vi "Listen.vi"(6 "Error":errorcluster, 7 "Actor":refnum<class "Actor Layer.lvclass">, 10 "Msg DVR":refnum<data-value>, 11 "Actor":T1) -> (3 "Actor":T1, 4 "Error":errorcluster, 5 "Actor":refnum<class "Actor Layer.lvclass">)   [LabVIEW 2020, in "jettl.lvlib"]
uses:
  jettl.lvlib
  Msg/Msg.lvclass
  Actor Layer/Actor Layer.lvclass
  Msg Attribs.ctl
  Origin.ctl
  Lifecycle.ctl
  Actor.ctl
  Children.ctl
  Actor Attribs.ctl
  Msg.ctl
  Post Setup.ctl
  Pre Setup.ctl
  Msg Set.ctl
  Layer Type.ctl
  Layer Attribs.ctl
  Layer Map.ctl
  Implemented Map.ctl
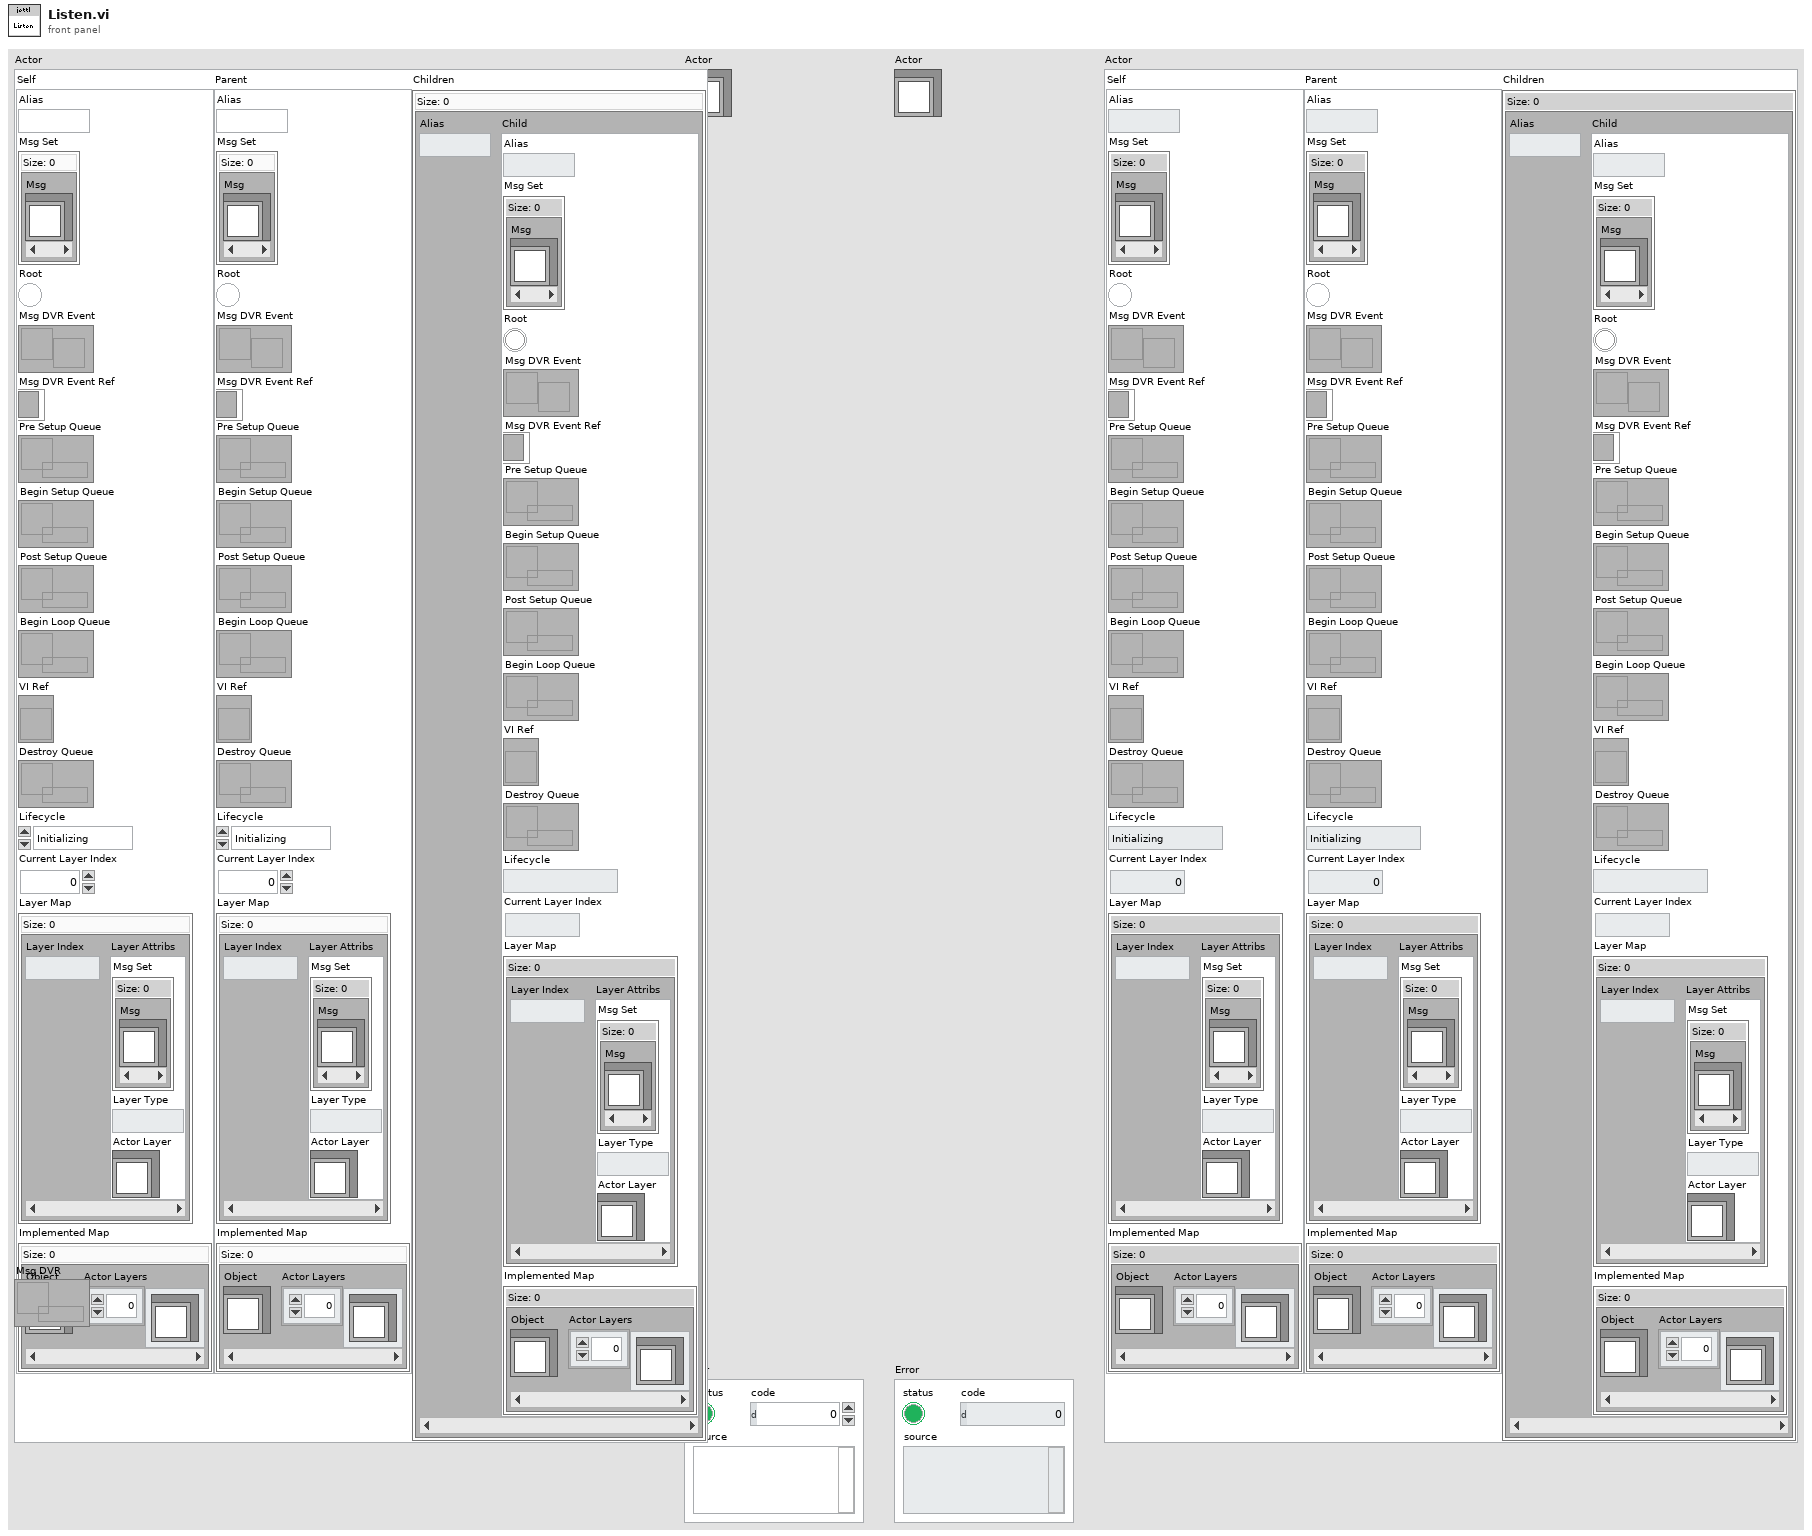
[diagram p1: front panel]
types:
  T1 = typedef "jettl.lvlib/Actor.ctl" = cluster{"Self":T2, "Parent":T2, "Children":T9}
  T2 = typedef "jettl.lvlib/Actor Attribs.ctl" = cluster{"Alias":string, "Msg Set":T3, "Root":bool, "Msg DVR Event":refnum<user-event>, "Msg DVR Event Ref":refnum<event-registration>, "Pre Setup Queue":refnum<queue>, "Begin Setup Queue":refnum<queue>, "Post Setup Queue":refnum<queue>, "Begin Loop Queue":refnum<queue>, "VI Ref":refnum<vi>, "Destroy Queue":refnum<queue>, "Lifecycle":T4, "Current Layer Index":i32, "Layer Map":T5, "Implemented Map":T8}
  T3 = typedef "jettl.lvlib/Msg Set.ctl" = set{refnum<class "Msg.lvclass">}
  T4 = typedef "jettl.lvlib/Lifecycle.ctl" = enum16{"Initializing", "Setting Up", "Starting", "Running", "Stopping", "Tearing Down", "Terminated"}
  T5 = typedef "jettl.lvlib/Layer Map.ctl" = map{i32, T6}
  T6 = typedef "jettl.lvlib/Layer Attribs.ctl" = cluster{"Msg Set":T3, "Layer Type":T7, "Actor Layer":refnum<class "Actor Layer.lvclass">}
  T7 = typedef "jettl.lvlib/Layer Type.ctl" = enum16{"Base", "InnerGlobal", "InnerLocal", "Outer"}
  T8 = typedef "jettl.lvlib/Implemented Map.ctl" = map{refnum<class>, refnum<class "Actor Layer.lvclass">[]}
  T9 = typedef "jettl.lvlib/Children.ctl" = map{string, T2}
  T10 = typedef "jettl.lvlib/Msg.ctl" = cluster{"Msg Attribs DVR":refnum<data-value>, "Msg Attribs":T11, "Msg":refnum<class "Msg.lvclass">, "Msg Default":refnum<class "Msg.lvclass">}
  T11 = typedef "jettl.lvlib/Msg Attribs.ctl" = cluster{"Priority":bool, "Listener Alias":string, "Teller Alias":string, "Teller Lifecycle":T4, "Teller Origin":T12, "Tell Absolute Time":timestamp, "Tell Relative Time":dbl, "Listen Absolute Time":timestamp, "Listen Relative Time":dbl}
  T12 = typedef "jettl.lvlib/Origin.ctl" = enum16{"Self", "Parent", "Child"}
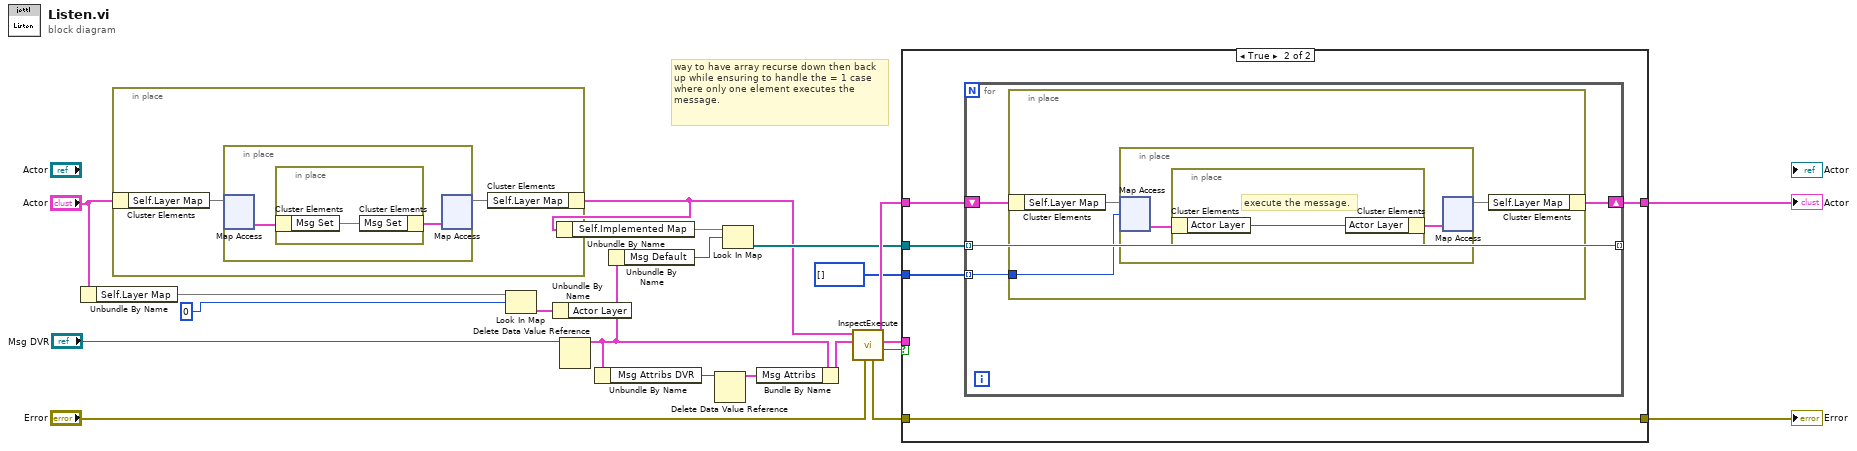
[diagram p0: block diagram]
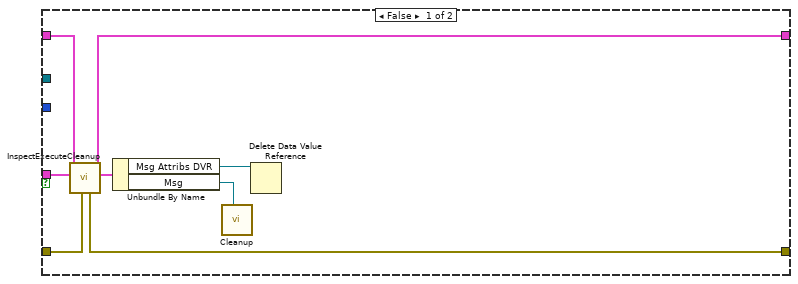
[diagram p2: hidden frame]
diagram:
  # "way to have array recurse down then back up while ensuring to handle the = 1 case where only one element executes the message."
  n1 = Unbundle By Name("Actor") -> ("Self.Layer Map"=w6:T5)
  n2 = in-place {
    n3 = in-place-cluster #1("Actor") -> ("Self.Layer Map"=w23:T5)
    n4 = in-place {
      n5 = in-place-map #2(w23) -> (w25:T6)  [unwired: 2 in, 1 out]
      n6 = in-place {
        n7 = in-place-cluster #3(w25) -> ("Msg Set"=w26:T3)
        n8 = in-place-cluster #3("Msg Set"=w26) -> (w24:T6)
      }
      n9 = in-place-map #2(w24) -> (w22:T5)  [unwired: 1 in, 2 out]
    }
    n10 = in-place-cluster #1("Self.Layer Map"=w22) -> (w2:T1)
  }
  n11 = Look In Map(map=w6, key=0) -> (value=w4:T6)  [unwired: 1 in, 1 out]
  n12 = Unbundle By Name(w4) -> ()  [unwired: 1 out]
  n13 = Unbundle By Name(w2) -> ("Self.Implemented Map"=w10:T8)
  n14 = Delete Data Value Reference(data value reference="Msg DVR") -> (data value=w9:T10)  [unwired: 1 in, 1 out]
  n15 = Unbundle By Name(w9) -> ("Msg Attribs DVR"=w13:refnum<data-value>)
  n16 = Unbundle By Name(w9) -> ("Msg Default"=w8:refnum<class "Msg.lvclass">)
  n17 = Delete Data Value Reference(data value reference=w13) -> (data value=w11:T11)  [unwired: 1 in, 1 out]
  n18 = Look In Map(map=w10, key=w8) -> (value=w7:refnum<class "Actor Layer.lvclass">[])  [unwired: 1 in, 1 out]
  n19 = Bundle By Name(cluster=w9, "Msg Attribs"=w11) -> (w12:T10)
  n20 = call-dynamic "InspectExecute.vi"("Error"="Error", "Msg"=w12, "Actor"=w2) -> ("Execute"=w16:bool, "Msg"=w15:T10, "Actor"=w17:T1, "Error"=w20:errorcluster)  [unwired: 4 in, 1 out]
  n21 = case shown="True" w16 {
    tunnel: w15 -> [w30 _]
    tunnel: [w33 w41] -> w21
    tunnel: w20 -> [w34 w41]
    tunnel: [w32 w38] -> w18
    tunnel: w17 -> [w31 w39]
    tunnel: w7 -> [_ w40]
    tunnel: i32[] [] -> [_ w37]
    frame False {
      n22 = call-dynamic "InspectExecuteCleanup.vi"("Error"=w34, "Msg"=w30, "Actor"=w31) -> ("Msg"=w29:T10, 3:"Actor"=w32:T1, "Error"=w33:errorcluster, 5:"Actor"=w36:refnum<class "Actor Layer.lvclass">, 7:"Actor"=w35:refnum<class "Actor Layer.lvclass">)  [unwired: 4 in]
      n23 = Unbundle By Name(w29) -> ("Msg Attribs DVR"=w27:refnum<data-value>, "Msg"=w28:refnum<class "Msg.lvclass">)
      n24 = call-dynamic "Cleanup.vi"("Msg"=w28) -> ()  [unwired: 11 in]
      n25 = Delete Data Value Reference(data value reference=w27) -> ()  [unwired: 1 in, 2 out]
    }
    frame True {
      n26 = for {
        tunnel: w40 -> [w45] mode=indexing
        shift-right: [w44] -> w38
        shift-left: w39 -> [w43]
        tunnel: [w45] -> _ mode=indexing
        tunnel: w37 -> [w42] mode=indexing
        n27 = in-place {
          in-place-border: w42 -> [w46]
          n28 = in-place-cluster #4(w43) -> ("Self.Layer Map"=w48:T5)
          n29 = in-place {
            n30 = in-place-map #5(w48, w46) -> (w50:T6)  [unwired: 1 in, 1 out]
            n31 = in-place {
              # "execute the message."
              n32 = in-place-cluster #6(w50) -> ("Actor Layer"=w51:refnum<class "Actor Layer.lvclass">)
              n33 = in-place-cluster #6("Actor Layer"=w51) -> (w49:T6)
            }
            n34 = in-place-map #5(w49) -> (w47:T5)  [unwired: 1 in, 2 out]
          }
          n35 = in-place-cluster #4("Self.Layer Map"=w47) -> (w44:T1)
        }
      }
    }
  }
  "Error" <- w21
  "Actor" <- w18
